vi "Set_FPGASimIO_Channel Data_5734.vi"(7 "Channel Name":string="Channel0", 8 "Error In":errorcluster, 11 "Data":i16) -> (0 "Error Out":errorcluster)   [LabVIEW 2012]
panel:
  in  "timeout in ms (-1)":i32=100
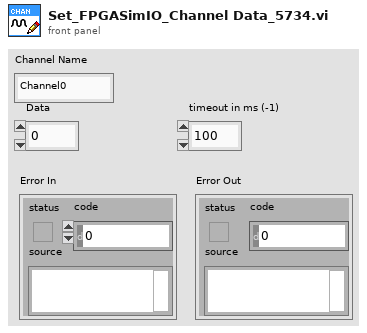
[diagram p1: front panel]
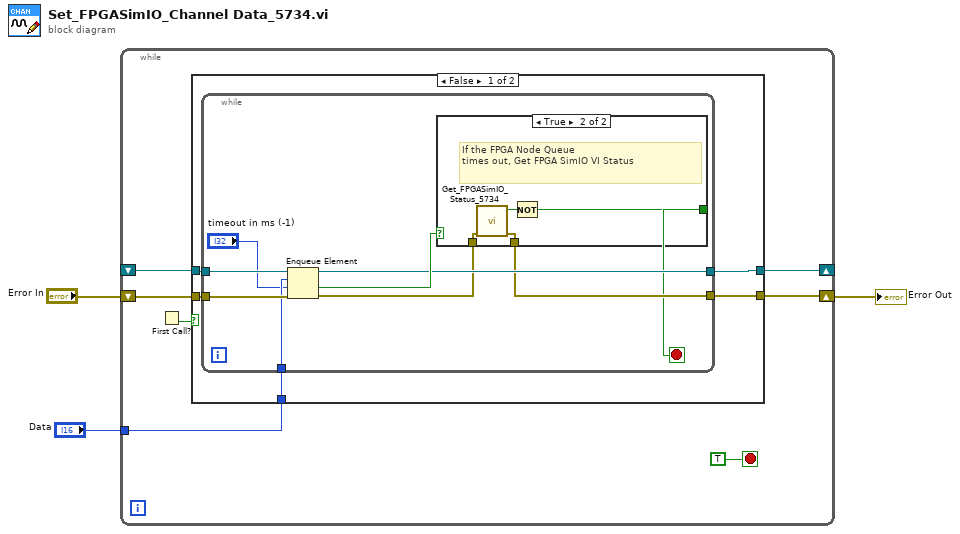
[diagram p0: block diagram]
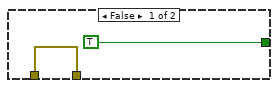
[diagram p2: hidden frame]
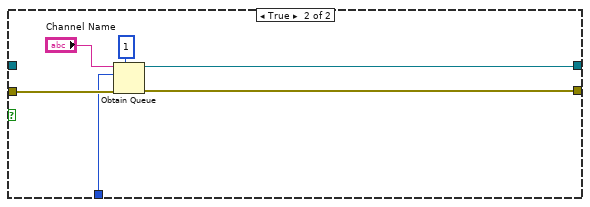
[diagram p3: hidden frame]
diagram:
  n1 = while {
    shift-right: [w7] -> w2
    shift-left: "Error In" -> [w9]
    shift-right: [w5] -> _
    shift-left: _ -> [w8]
    tunnel: "Data" -> [w6]
    stop <- TRUE stop-if-true
    n2 = First Call?() -> (First Call?: T/F=w10:bool)
    n3 = case shown="False" w10 {
      tunnel: [w12 w33] -> w5
      tunnel: [w11 w35] -> w7
      tunnel: w8 -> [w15 _]
      tunnel: w9 -> [w14 w34]
      tunnel: w6 -> [w13 w31]
      frame False {
        n4 = while {
          tunnel: w15 -> [w24]
          tunnel: w14 -> [w23]
          tunnel: w13 -> [w22]
          tunnel: [w19] -> w12
          tunnel: [w17] -> w11
          stop <- w16 stop-if-true
          n5 = Enqueue Element(queue=w24, element=w22, timeout in ms (-1)="timeout in ms (-1)", error in (no error)=w23) -> (queue out=w19:refnum<queue>, timed out?=w20:bool, error out=w18:errorcluster)
          n6 = case shown="True" w20 {
            tunnel: w18 -> [w26 w30]
            tunnel: [w26 w29] -> w17
            tunnel: [TRUE w27] -> w16
            frame False {
            }
            frame True {
              # "If the FPGA Node Queue \ntimes out, Get FPGA SimIO VI Status"
              n7 = call "Get_FPGASimIO_Status_5734.vi"("Error In"=w30) -> ("Error Out"=w29:errorcluster, "Sim IO FPGA Status"=w28:bool)  [unwired: 9 in]
              n8 = Not(x=w28) -> (.not. x?=w27:bool)
            }
          }
        }
      }
      frame True {
        n9 = Obtain Queue(max queue size (-1, unlimited)=1, name (unnamed)="Channel Name", element data type=w31, error in (no error)=w34) -> (queue out=w33:refnum<queue>, error out=w35:errorcluster)  [unwired: 1 in, 1 out]
      }
    }
  }
  "Error Out" <- w2
